vi "Subtract headings.vi"(1 "Old Heading":dbl, 2 "New Heading":dbl) -> (0 "Heading Change":dbl)   [LabVIEW 2011]
doc: "Finds the shortest heading difference between two headings (-180 to 180). Note that it assumes that the input headings are between 0 and 360."
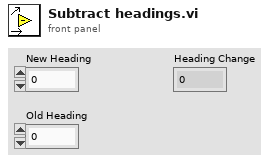
[diagram p1: front panel]
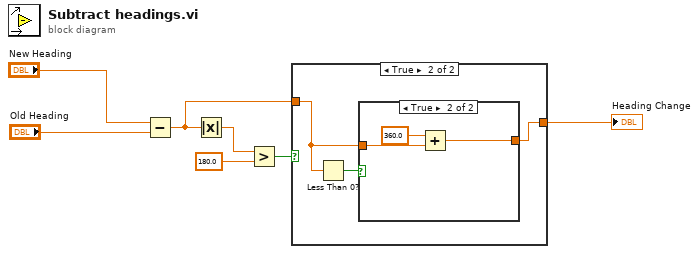
[diagram p0: block diagram]
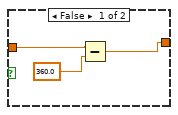
[diagram p3: hidden frame]
diagram:
  n1 = Subtract(x="New Heading", y="Old Heading") -> (x-y=w6:dbl)
  n2 = Absolute Value(x=w6) -> (abs(x)=w4:dbl)
  n3 = Greater?(x=w4, y=180.0) -> (0:w5:bool)
  n4 = case shown="True" w5 {
    tunnel: w6 -> [w8 w10]
    tunnel: [w8 w9] -> w7
    frame False {
    }
    frame True {
      n5 = Less Than 0?(x=w10) -> (x < 0?=w11:bool)
      n6 = case shown="True" w11 {
        tunnel: w10 -> [w14 w16]
        tunnel: [w12 w15] -> w9
        frame False {
          n7 = Subtract(x=w14, y=360.0 ("x")) -> (x-y=w12:dbl)
        }
        frame True {
          n8 = Add(x=360.0, y=w16) -> (x+y=w15:dbl)
        }
      }
    }
  }
  "Heading Change" <- w7
